vi "Read.vi"(8 "error in (no error)":errorcluster, 9 "Variant":variant, 11 "AK RS232 in":refnum<class "AK RS-xxx.lvclass">) -> (0 "error out":errorcluster, 2 "String":string, 3 "AK RS232 out":refnum<class "AK RS-xxx.lvclass">)   [LabVIEW 2019, in "Protocols.lvlib" / "AK RS-xxx.lvclass"]
uses:
  AK RS-xxx.lvclass
  Protocol Parent/Methods/Read Parameter.ctl
  AK RS-xxx.lvclass/AK RS-xxx.ctl
  Data Access/Read Current Command Code.vi
  <vilib>/Utility/error.llb/Error Cluster From Error Code.vi
  RS-xxx/RS-xxx.lvclass
  Protocols.lvlib
  Protocol Parent/Protocol Parent.lvclass
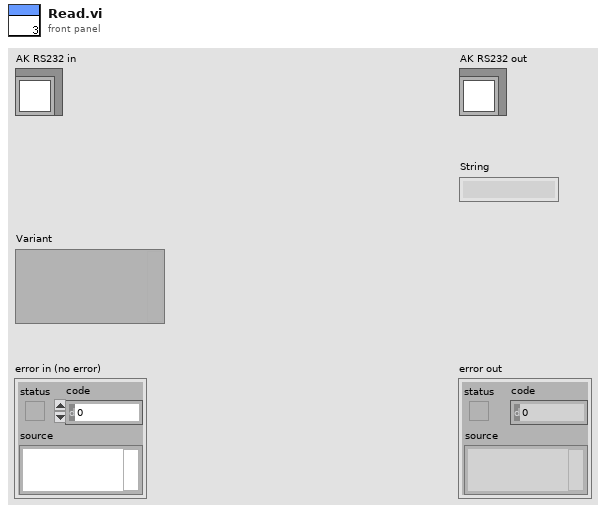
[diagram p1: front panel]
types:
  T1 = typedef "Protocols.lvlib/Protocol Parent.lvclass/Read Parameter.ctl" = cluster{"Wait Type":enum16{"Byte Count", "Wait sec"}, "Wait Value":dbl}
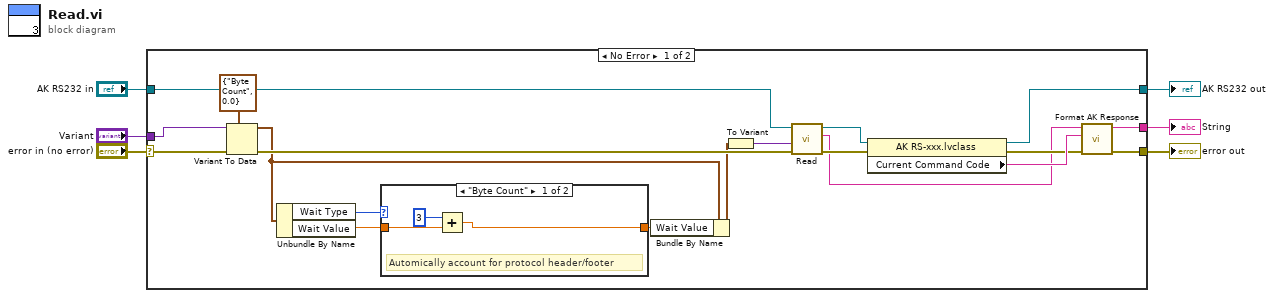
[diagram p0: block diagram]
diagram:
  n1 = case shown="No Error" "error in (no error)" {
    selector: "error in (no error)" -> [w14 w31]
    tunnel: "Variant" -> [w15 _]
    tunnel: "AK RS232 in" -> [w25 w30]
    tunnel: [w22 w30] -> w4
    tunnel: [w20 _] -> w3
    tunnel: [w18 w31] -> w2
    frame No Error {
      n2 = Variant To Data(error in=w14, type=T1 {"Wait Type"=enum."Byte Count", "Wait Value"=0.0} ("Read Parameter"), Variant=w15) -> (data=w10:T1, error out=w13:errorcluster)
      n3 = Unbundle By Name(w10) -> ("Wait Type"=w12:enum16{"Byte Count", "Wait sec"}, "Wait Value"=w11:dbl)
      n4 = case shown="\"Byte Count\"" w12 {
        tunnel: w11 -> [w28 w29]
        tunnel: [w26 w29] -> w9
        frame "Byte Count" {
          # "Automically account for protocol header/footer"
          n5 = Add(x=3, y=w28) -> (x+y=w26:dbl)
        }
        frame "Wait sec" {
        }
      }
      n6 = Bundle By Name(cluster=w10, "Wait Value"=w9) -> (w7:T1)
      n7 = To Variant(anything=w7) -> (Variant=w8:variant)
      n8 = call-parent "Read.vi"("error in (no error)"=w13, "Variant"=w8, "RS232 in"=w25) -> ("error out"=w24:errorcluster, "String"=w17:string, "RS232 out"=w23:refnum<class "AK RS-xxx.lvclass">)  [unwired: 6 in]
      n9 = property class="AK RS-xxx.lvclass"(reference=w23, error in=w24) -> (reference out=w22:refnum<class "AK RS-xxx.lvclass">, error out=w19:errorcluster, "Current Command Code"=w21:string)
      n10 = call "Format AK Response.vi"("error in (no error)"=w19, "Current Command Code"=w21, "Response"=w17) -> ("error out"=w18:errorcluster, "Data"=w20:string)  [unwired: 7 in]
    }
    frame Error {
    }
  }
  "error out" <- w2
  "AK RS232 out" <- w4
  "String" <- w3
